vi "ZDataVIS_Decimate+Fill_Intensity_Plot.vi"(6 "fake point value":dbl, 7 "Voffset -2T":dbl, 8 "error in (no error)":errorcluster, 9 "Step Info":cluster{"X Low":dbl, "X High":dbl, "X Step":dbl}={"X Low"=-0.1, "X High"=0.1, "X Step"=4e-05} {"X Step" format="%#_6p"; "X High" format="%#_6p"; "X Low" format="%#_6p"}, 10 "X and Y Arrays to decimate":T3(array[cluster]), 11 "State Wire IN":T1={"Core"={"Current VI Reference"=refnum, "Close Panel on Exit?"=FALSE}, "Sweep Data Cluster"={"Vfast"=[], "Vslow"=[], "Vslowest"=[], "Comments"="", "Scan names"=[]}, "Cursor Info"={"Fast Index"=[], "Slow Index"=0.0, "Slow Indices"=[], "Raw Cursor Position"={"X"=0.0, "Y"=0.0}, "Field / temp"=0}, "Scan names"=[], "Data DVR"=refnum, "Arr of Y arrays (intensity info)"=[], "Decimated X values"=[], "X Step Info"={"X Low"=-0.1, "X High"=0.1, "X Step"=4e-05}, "Voffset -2T"=0.0} {"X Step Info"."X Step" format="%#_6p"; "X Step Info"."X High" format="%#_6p"; "X Step Info"."X Low" format="%#_6p"}) -> (0 "error out":errorcluster, 1 "Decimated X values":dbl[](array[numeric]), 2 "Arr of Y arrays (intensity info)":dbl[][](array[numeric]), 3 "State Wire OUT":T1={"Core"={"Current VI Reference"=refnum, "Close Panel on Exit?"=FALSE}, "Sweep Data Cluster"={"Vfast"=[], "Vslow"=[], "Vslowest"=[], "Comments"="", "Scan names"=[]}, "Cursor Info"={"Fast Index"=[], "Slow Index"=0.0, "Slow Indices"=[], "Raw Cursor Position"={"X"=0.0, "Y"=0.0}, "Field / temp"=0}, "Scan names"=[], "Data DVR"=refnum, "Arr of Y arrays (intensity info)"=[], "Decimated X values"=[], "X Step Info"={"X Low"=-0.1, "X High"=0.1, "X Step"=4e-05}, "Voffset -2T"=0.0} {"X Step Info"."X Step" format="%#_6p"; "X Step Info"."X High" format="%#_6p"; "X Step Info"."X Low" format="%#_6p"})   [LabVIEW 2016]
uses:
  ZDataVIS_StateWire.ctl
  <vilib>/Utility/miscctls.llb/LVPointDoubleTypeDef.ctl
panel:
  # "cursor x"
  # "cursor y"
  # "cursor x"
  # "cursor y"
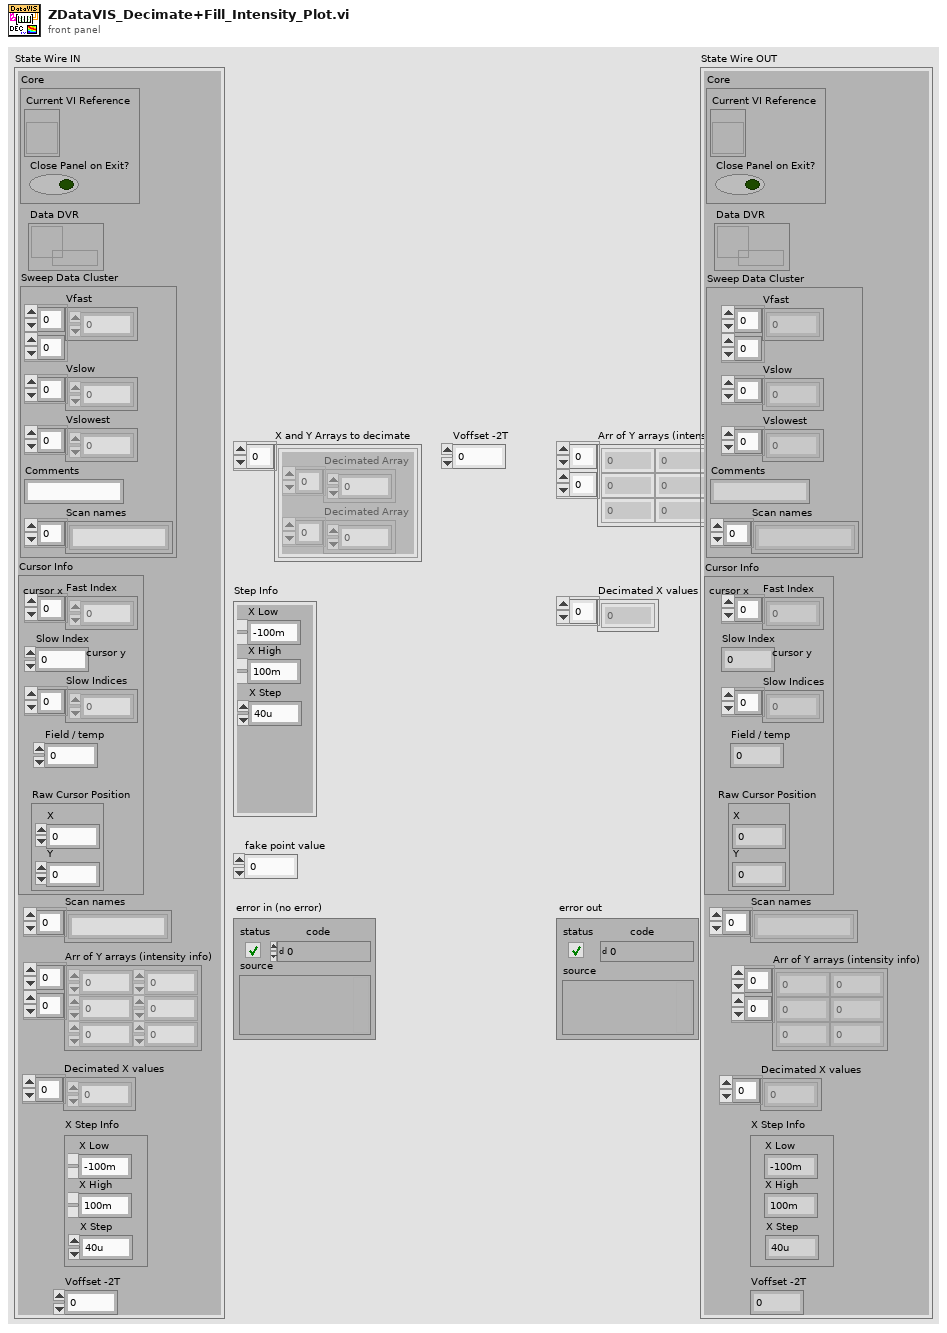
[diagram p1: front panel]
types:
  T1 = typedef "ZDataVIS_StateWire.ctl" = cluster{"Core":cluster{"Current VI Reference":refnum<vi>, "Close Panel on Exit?":bool}, "Sweep Data Cluster":cluster{"Vfast":dbl[][], "Vslow":dbl[], "Vslowest":dbl[], "Comments":string, "Scan names":string[]}, "Cursor Info":cluster{"Fast Index":dbl[], "Slow Index":dbl, "Slow Indices":dbl[], "Raw Cursor Position":T2, "Field / temp":i32}, "Scan names":string[], "Data DVR":refnum<data-value>, "Arr of Y arrays (intensity info)":dbl[][], "Decimated X values":dbl[], "X Step Info":cluster{"X Low":dbl, "X High":dbl, "X Step":dbl}, "Voffset -2T":dbl}
  T2 = typedef "LVPointDoubleTypeDef.ctl" = cluster{"X":dbl, "Y":dbl}
  T3 = cluster{"Decimated Array":dbl[], "Decimated Array":dbl[]}[]
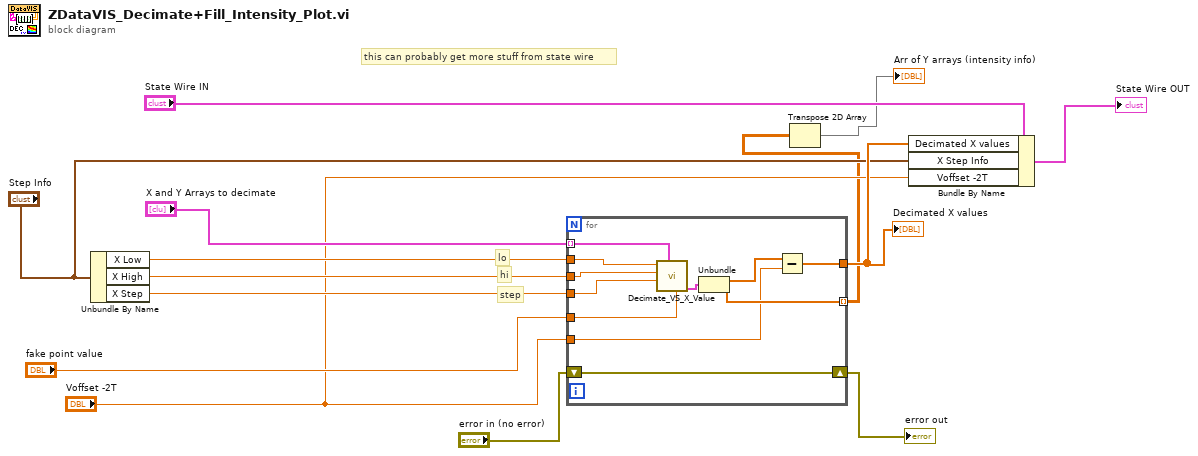
[diagram p0: block diagram]
diagram:
  # "this can probably get more stuff from state wire"
  # "lo"
  # "hi"
  # "step"
  n1 = Unbundle By Name("Step Info") -> ("X Low"=w10:dbl, "X High"=w9:dbl, "X Step"=w8:dbl)
  n2 = for {
    tunnel: [w24] -> w5
    tunnel: "X and Y Arrays to decimate" -> [w19] mode=indexing
    tunnel: [w23] -> w2 mode=indexing
    tunnel: w10 -> [w22]
    tunnel: w9 -> [w21]
    tunnel: w8 -> [w20]
    tunnel: "Voffset -2T" -> [w17]
    tunnel: "fake point value" -> [w16]
    shift-right: [w15] -> w12
    shift-left: "error in (no error)" -> [w15]
    n3 = call <userlib>:"Decimate_VS_X_Value.vi"("fake point value"=w16, "XY Graph kind 1"=w19, "X Step"=w20, "X High"=w21, "X Low"=w22) -> ("Interpreted"=w18:cluster{dbl[], dbl[]})  [unwired: 5 in, 1 out]
    n4 = Unbundle(w18) -> (w25:dbl[], w23:dbl[])
    n5 = Subtract(x=w25, y=w17) -> (x-y=w24:dbl[])
  }
  "Decimated X values" <- w5
  "error out" <- w12
  n6 = Transpose 2D Array(2D array=w2) -> (transposed array=→"Arr of Y arrays (intensity info)":dbl[][])
  n7 = Bundle By Name(cluster="State Wire IN", "Decimated X values"=w5, "X Step Info"="Step Info", "Voffset -2T"="Voffset -2T") -> (→"State Wire OUT":T1)
